vi "Build Driver Settings Mappings.vi"(8 "error in (no error)":errorcluster, 11 "HMC8043 in":refnum<class "HMC8043.lvclass">) -> (0 "error out":errorcluster, 3 "HMC8043 out":refnum<class "HMC8043.lvclass">)   [LabVIEW 2023, in "HAF.lvlib" / "HMC8043.lvclass"]
uses:
  HMC8043.lvclass
  HMC8043.lvclass/HMC8043.ctl
  Driver/Driver.lvclass
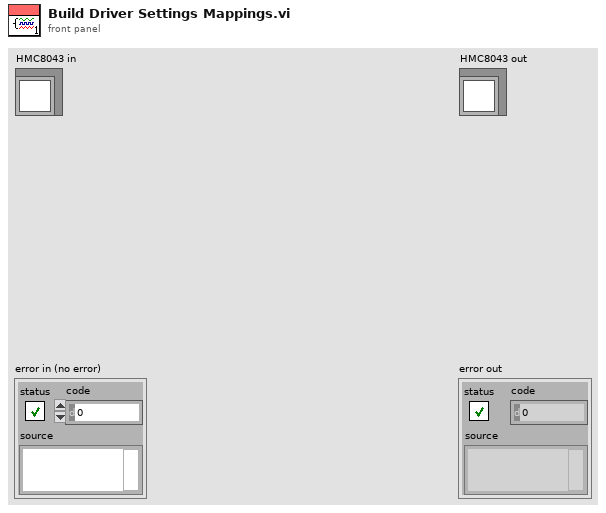
[diagram p1: front panel]
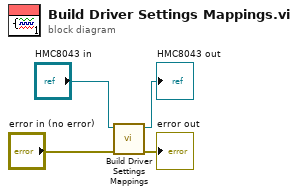
[diagram p0: block diagram]
diagram:
  n1 = call-parent "Build Driver Settings Mappings.vi"("error in (no error)"="error in (no error)", "Driver in"="HMC8043 in") -> ("error out"=→"error out":errorcluster, "Driver out"=→"HMC8043 out":refnum<class "HMC8043.lvclass">)  [unwired: 8 in]
